vi "Frequency.vi"(8 "Samples per calculation":dbl, 11 "Input waveform":waveform(dbl)) -> (3 "Frequency waveform":waveform(dbl))   [LabVIEW 2019]
uses:
  <vilib>/measure/mascope.llb/Pulse Measurements 1 chan.vi
  <vilib>/measure/NI_MAPro.lvlib
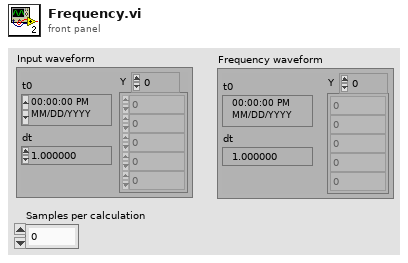
[diagram p1: front panel]
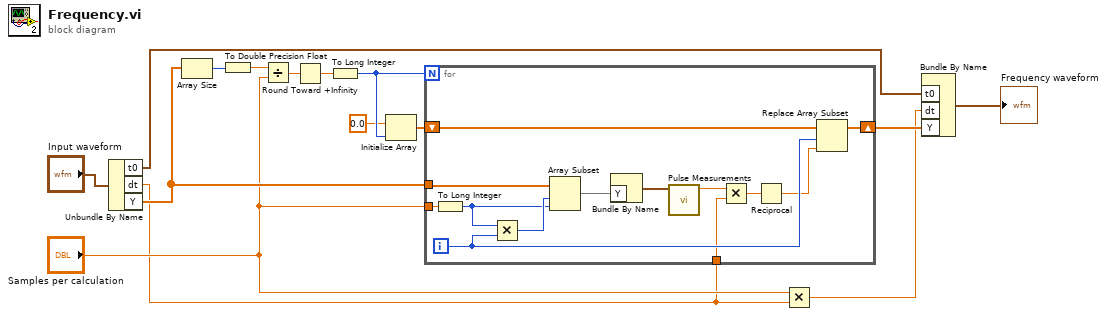
[diagram p0: block diagram]
diagram:
  n1 = Unbundle By Name("Input waveform") -> ("t0"=w4:timestamp, "dt"=w1:dbl, "Y"=w10:dbl[])
  n2 = Array Size(array=w10) -> (size(s)=w11:i32)
  n3 = To Double Precision Float(number=w11) -> (double precision float=w12:dbl)
  n4 = Divide(x=w12, y="Samples per calculation") -> (x/y=w14:dbl)
  n5 = Round Toward +Infinity(x=w14) -> (ceil(x): smallest int >= x=w13:dbl)
  n6 = To Long Integer(number=w13) -> (32bit integer=w9:i32)
  n7 = Initialize Array(0.0 ("element"), w9) -> (w8:dbl[])
  n8 = for {
    N: w9 -> [_]
    tunnel: w10 -> [w27]
    tunnel: "Samples per calculation" -> [w25]
    shift-right: [w20] -> w5
    shift-left: w8 -> [w22]
    tunnel: w1 -> [w18]
    i -> [w21]
    n9 = To Long Integer(number=w25) -> (32bit integer=w23:i32)
    n10 = Multiply(x=w23, y=w21) -> (x*y=w24:i32)
    n11 = Array Subset(array=w27, index=w24, length=w23) -> (w26:dbl[])
    n12 = Bundle By Name("Y"=w26) -> (w28:waveform(dbl))  [unwired: 1 in]
    n13 = call-poly <vilib>:"Pulse Measurements.vi"("signal in"=w28) -> ("period"=w19:dbl)  [unwired: 6 in, 4 out]
    n14 = Multiply(x=w19, y=w18) -> (x*y=w17:dbl)
    n15 = Reciprocal(x=w17) -> (1/x=w16:dbl)
    n16 = Replace Array Subset(array=w22, new element=w16, index=w21) -> (w20:dbl[])
  }
  n17 = Multiply(x="Samples per calculation", y=w1) -> (x*y=w2:dbl)
  n18 = Bundle By Name("t0"=w4, "dt"=w2, "Y"=w5) -> (→"Frequency waveform":waveform(dbl))  [unwired: 1 in]
